vi "p2.vi"() -> ()   [LabVIEW 2023, in "d16.lvlib"]
uses:
  d16.lvlib
  AOC/AOC.lvlib
panel:
  in  "Example":string=".|...\\....\n|.-.\\.....\n.....|-...\n........|.\n..........\n.........\\\n..../.\\\\..\n.-.-/..|..\n.|....-|.\\\n..//.|...."
  in  "Example":bool=TRUE
  out "Answer":u64=15
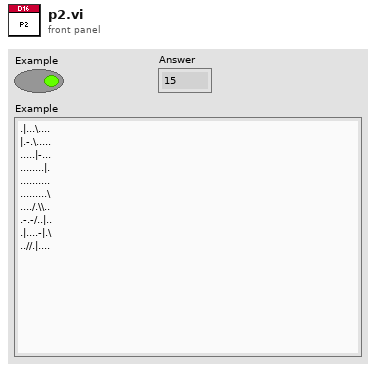
[diagram p1: front panel]
types:
  T1 = cluster{"position":cluster{"x":i32, "y":i32}, "direction":string}
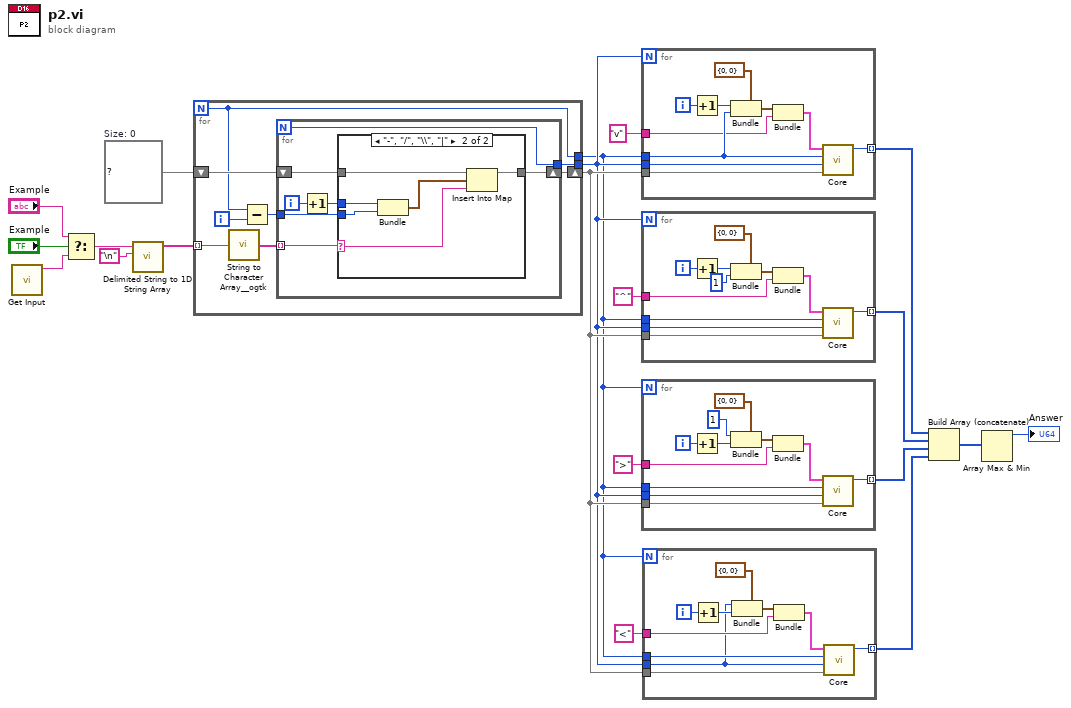
[diagram p0: block diagram]
diagram:
  w14 = map{cluster{i32, i32}, string} {}  # Size: 0
  n1 = call "Get Input.vi"() -> ("Input"=w20:string)  [unwired: 11 in]
  n2 = Select(t="Example", s="Example", f=w20) -> (s? t:f=w19:string)
  n3 = call <vilib>:"Delimited String to 1D String Array.vi"("delimiter"="\n", "delimited string"=w19) -> ("string array"=w15:string[])  [unwired: 9 in]
  n4 = for {
    N -> [w22]
    tunnel: w15 -> [w28] mode=indexing
    shift-right: [w24] -> w9
    shift-left: w14 -> [w25]
    tunnel: [w22] -> w1
    tunnel: [w23] -> w2
    i -> [w26]
    n5 = call <userlib>:"String to Character Array__ogtk.vi"("Input String"=w28) -> ("Character Array"=w27:string[])
    n6 = Subtract(x=w22, y=w26) -> (x-y=w21:i32)
    n7 = for {
      N -> [w30]
      tunnel: w27 -> [w35] mode=indexing
      tunnel: w21 -> [w33]
      shift-right: [w31] -> w24
      shift-left: w25 -> [w32]
      tunnel: [w30] -> w23
      i -> [w34]
      n8 = Increment(x=w34) -> (x+1=w29:i32)
      n9 = case shown="\"-\", \"/\", \"\\\\\", \"|\"" w35 {
        selector: w35 -> [_ w40]
        tunnel: w29 -> [_ w42]
        tunnel: w33 -> [_ w41]
        tunnel: w32 -> [w36 w39]
        tunnel: [w36 w38] -> w31
        frame Default {
        }
        frame "-", "/", "\\", "|" {
          n10 = Bundle(w42, w41) -> (w37:cluster{i32, i32})  [unwired: 1 in]
          n11 = Insert Into Map(map in=w39, key=w37, value=w40) -> (map out=w38:map{cluster{i32, i32}, string})  [unwired: 2 out]
        }
      }
    }
  }
  n12 = for {
    N: w2 -> [_]
    tunnel: w2 -> [w52]
    tunnel: [w51] -> w8 mode=indexing
    tunnel: w1 -> [w50]
    tunnel: "v" ("direction") -> [w47]
    tunnel: w9 -> [w45]
    i -> [w44]
    n13 = Increment(x=w44) -> (x+1=w43:i32)
    n14 = Bundle(cluster=cluster{"x":i32, "y":i32} {"x"=0, "y"=0} ("position"), "x"=w43, "y"=w50) -> (w48:cluster{"x":i32, "y":i32})
    n15 = Bundle("position"=w48, "direction"=w47) -> (w46:T1)  [unwired: 1 in]
    n16 = call "Core.vi"("Mirrors& Splitters"=w45, "ySize"=w52, "xSize"=w50, "Initial Lazer"=w46) -> ("Number Energized"=w51:i32)  [unwired: 7 in]
  }
  n17 = for {
    N: w2 -> [_]
    tunnel: w2 -> [w63]
    tunnel: [w62] -> w7 mode=indexing
    tunnel: w1 -> [w61]
    tunnel: "^" ("direction") -> [w58]
    tunnel: w9 -> [w56]
    i -> [w55]
    n18 = Increment(x=w55) -> (x+1=w54:i32)
    n19 = Bundle(cluster=cluster{"x":i32, "y":i32} {"x"=0, "y"=0} ("position"), "x"=w54, "y"=1) -> (w59:cluster{"x":i32, "y":i32})
    n20 = Bundle("position"=w59, "direction"=w58) -> (w57:T1)  [unwired: 1 in]
    n21 = call "Core.vi"("Mirrors& Splitters"=w56, "ySize"=w63, "xSize"=w61, "Initial Lazer"=w57) -> ("Number Energized"=w62:i32)  [unwired: 7 in]
  }
  n22 = for {
    N: w1 -> [_]
    tunnel: w2 -> [w74]
    tunnel: [w73] -> w6 mode=indexing
    tunnel: w1 -> [w72]
    tunnel: ">" ("direction") -> [w69]
    tunnel: w9 -> [w67]
    i -> [w66]
    n23 = Increment(x=w66) -> (x+1=w64:i32)
    n24 = Bundle(cluster=cluster{"x":i32, "y":i32} {"x"=0, "y"=0} ("position"), "x"=1 ("y"), "y"=w64) -> (w70:cluster{"x":i32, "y":i32})
    n25 = Bundle("position"=w70, "direction"=w69) -> (w68:T1)  [unwired: 1 in]
    n26 = call "Core.vi"("Mirrors& Splitters"=w67, "ySize"=w74, "xSize"=w72, "Initial Lazer"=w68) -> ("Number Energized"=w73:i32)  [unwired: 7 in]
  }
  n27 = for {
    N: w1 -> [_]
    tunnel: w2 -> [w75]
    tunnel: [w84] -> w5 mode=indexing
    tunnel: w1 -> [w83]
    tunnel: "<" ("direction") -> [w80]
    tunnel: w9 -> [w78]
    i -> [w77]
    n28 = Increment(x=w77) -> (x+1=w76:i32)
    n29 = Bundle(cluster=cluster{"x":i32, "y":i32} {"x"=0, "y"=0} ("position"), "x"=w75, "y"=w76) -> (w81:cluster{"x":i32, "y":i32})
    n30 = Bundle("position"=w81, "direction"=w80) -> (w79:T1)  [unwired: 1 in]
    n31 = call "Core.vi"("Mirrors& Splitters"=w78, "ySize"=w75, "xSize"=w83, "Initial Lazer"=w79) -> ("Number Energized"=w84:i32)  [unwired: 7 in]
  }
  n32 = Build Array (concatenate)(w8, w7, w6, w5) -> (w4:i32[])
  n33 = Array Max & Min(array=w4) -> (max value=→"Answer":i32)  [unwired: 3 out]
